vi "Monitor Demo.vi"() -> ()   [LabVIEW 2022 SP3]
uses:
  Flex/Instantiate.vi
  Flex/Flex.lvlib
panel:
  out "Stalled":bool
  out "Actual":u32
  out "Lossless 50mS":dbl(graph)
  out "Lossless 20mS":dbl(graph)
  out "Lossless 5mS":dbl(graph)
  in  "Stop":bool
  in  "Period mS":u32=20
  out "Buffers":dbl[](array[slide]) scale=0.0..1.0
  in  "Slide":dbl(slide) scale=0.0..10.0
  out "Count":i32[](array[numeric])
  # "Producer"
  # "The order of consumers can be random in these indicators"
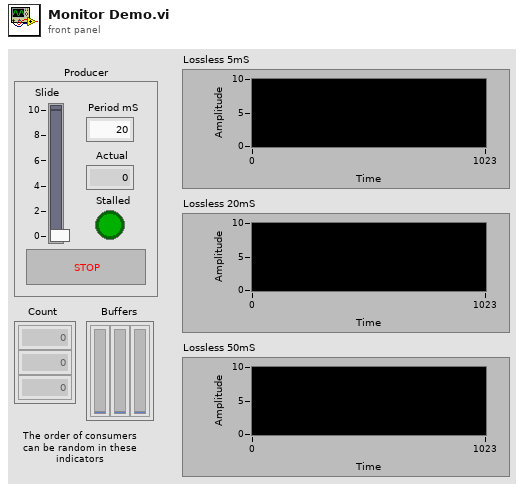
[diagram p1: front panel]
types:
  T1 = typedef "Flex.lvlib/))Channel.ctl" = refnum<queue>
  T2 = typedef "Flex.lvlib/Element.ctl" = dbl
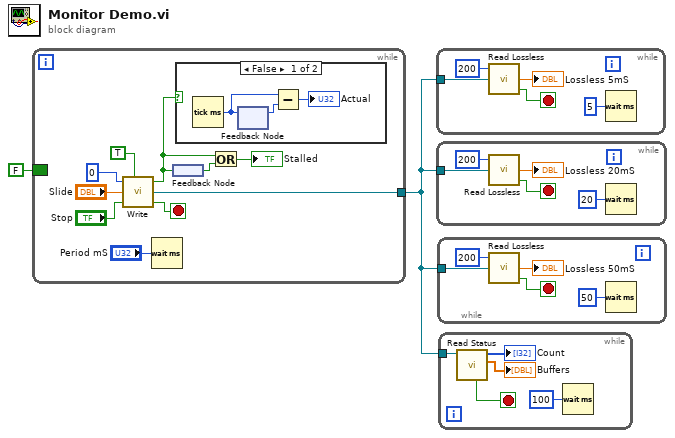
[diagram p0: block diagram]
diagram:
  n1 = while {
    tunnel: [w9] -> w2
    border: FALSE ("Timed Out?") -> [_]
    stop <- w5 stop-if-true
    n2 = call "Write.vi"("Timeout mS (-1)"=0, "Synchronous (T)"=TRUE, "element"="Slide", "Close? (F)"="Stop") -> ("Timed Out?"=w4:bool, "channel"=w9:T1, "Closed?"=w5:bool)  [unwired: 3 in]
    n3 = Wait (ms)(milliseconds to wait="Period mS") -> ()  [unwired: 1 out]
    n4 = feedback #1() -> (w7:bool)
    n5 = feedback-in #1(w4) -> ()
    n6 = case shown="False" w4 {
      frame False {
        n7 = Tick Count (ms)() -> (millisecond timer value=w14:u32)
        n8 = feedback #2() -> (w13:u32)  [unwired: 1 in]
        n9 = feedback-in #2(w14) -> ()
        n10 = Subtract(x=w14, y=w13) -> (x-y=→"Actual":u32)
      }
      frame True {
      }
    }
    n11 = Or(x=w4, y=w7) -> (x .or. y?=→"Stalled":bool)
  }
  n12 = while {
    tunnel: w2 -> [w20]
    stop <- w16 stop-if-true
    n13 = call "Read Lossless.vi"("Depth (Unlimited)"=200, "FlexChannel"=w20) -> ("Element"=→"Lossless 5mS":T2, "Closed?"=w16:bool)  [unwired: 5 in, 1 out]
    n14 = Wait (ms)(milliseconds to wait=u32 5) -> ()  [unwired: 1 out]
  }
  n15 = while {
    tunnel: w2 -> [w25]
    stop <- w21 stop-if-true
    n16 = call "Read Lossless.vi"("Depth (Unlimited)"=200, "FlexChannel"=w25) -> ("Element"=→"Lossless 20mS":T2, "Closed?"=w21:bool)  [unwired: 5 in, 1 out]
    n17 = Wait (ms)(milliseconds to wait=u32 20) -> ()  [unwired: 1 out]
  }
  n18 = while {
    tunnel: w2 -> [w30]
    stop <- w26 stop-if-true
    n19 = call "Read Lossless.vi"("Depth (Unlimited)"=200, "FlexChannel"=w30) -> ("Element"=→"Lossless 50mS":T2, "Closed?"=w26:bool)  [unwired: 5 in, 1 out]
    n20 = Wait (ms)(milliseconds to wait=u32 50) -> ()  [unwired: 1 out]
  }
  n21 = while {
    tunnel: w2 -> [w34]
    stop <- w33 stop-if-true
    n22 = call "Read Status.vi"("channel"=w34) -> ("Usage Ratio"=→"Buffers":dbl[], "Queued Count"=→"Count":i32[], "Closed?"=w33:bool)  [unwired: 2 in, 6 out]
    n23 = Wait (ms)(milliseconds to wait=u32 100) -> ()  [unwired: 1 out]
  }
